vi "FlatToRichni_measurementlink_sessionmanagement_v1_ReserveAllRegisteredSessionsRequest_AnnotationsEntry.vi"(5 "OutputClusterType":T1, 11 "InputCluster":T2) -> (3 "OutputCluster":T1)   [LabVIEW 2021, in "ni.measurementlink.sessionmanagement.v1.api.lvlib"]
uses:
  ni.measurementlink.sessionmanagement.v1.api.lvlib
  ni_measurementlink_sessionmanagement_v1_ReserveAllRegisteredSessionsRequest_AnnotationsEntry_Flat.ctl
  ni_measurementlink_sessionmanagement_v1_ReserveAllRegisteredSessionsRequest_AnnotationsEntry.ctl
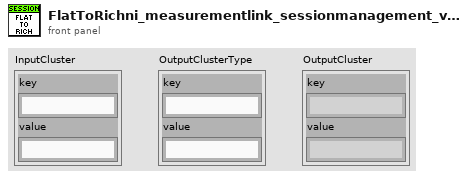
[diagram p1: front panel]
types:
  T1 = typedef "ni.measurementlink.sessionmanagement.v1.api.lvlib/ni_measurementlink_sessionmanagement_v1_ReserveAllRegisteredSessionsRequest_AnnotationsEntry.ctl" = cluster{"key":string, "value":string}
  T2 = typedef "ni.measurementlink.sessionmanagement.v1.api.lvlib/ni_measurementlink_sessionmanagement_v1_ReserveAllRegisteredSessionsRequest_AnnotationsEntry_Flat.ctl" = cluster{"key":string, "value":string}
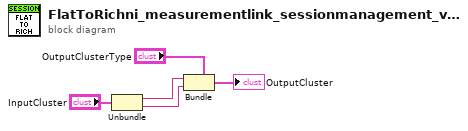
[diagram p0: block diagram]
diagram:
  n1 = Unbundle "Unbundle"("InputCluster") -> ("key"=w2:string, "value"=w1:string)
  n2 = Bundle "Bundle"(cluster="OutputClusterType", "key"=w2, "value"=w1) -> (→"OutputCluster":T1)
